vi "Locate SCM Breakdown.vi"(0 "Signals":waveform(dbl)[](array[waveform]), 7 "Offset (µs)":dbl format="%#_13g", 9 "Duration (µs)":dbl format="%#_13g", 11 "error in (no error)":errorcluster, 13 "Microphone Coordinates (cm, rad)":cluster{"r":dbl, "theta":dbl}[](array[cluster])) -> (4 "Coordinates (cm, rad, cm)":cluster{"r":sgl, "theta":sgl, "z":sgl}[](array[cluster]), 8 "Upstream/Downstream Delay (s)":dbl, 15 "error out":errorcluster)   [LabVIEW 2013]
uses:
  <vilib>/Analysis/2dsp.llb/1D Cross Correlation (DBL).vi
  <vilib>/Waveform/WDTOps.llb/WDT Get Waveform Subset DBL.vi
  <vilib>/Waveform/WDTOps.llb/WDT Index Channel DBL.vi
  <vilib>/Analysis/NI_AALPro.lvlib
  Breakdown Acoustics Controls/Breakdown Acoustics Controls.lvlib
panel:
  out "Sampling Rate":u16
  out "Array":i32[](array[numeric])
  out "Source Signals Correlation":dbl[](graph)
  out "Shifted Source Signals":dbl[][](graph)
  out "Downstream Signals":waveform(dbl)[](graph)
  out "Upstream Signals":waveform(dbl)[](graph)
  out "Duration (S)":dbl
  out "Offset (S)":dbl
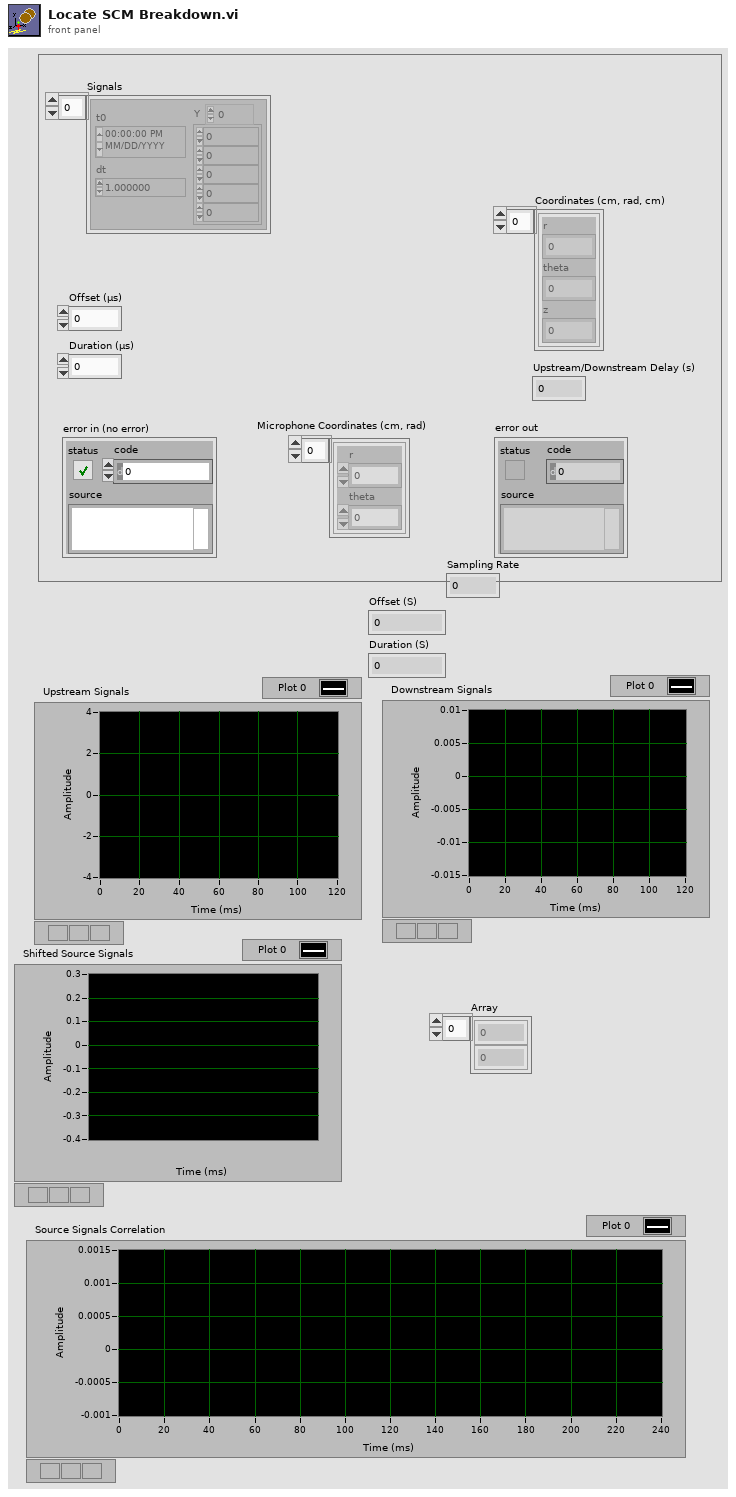
[diagram p1: front panel]
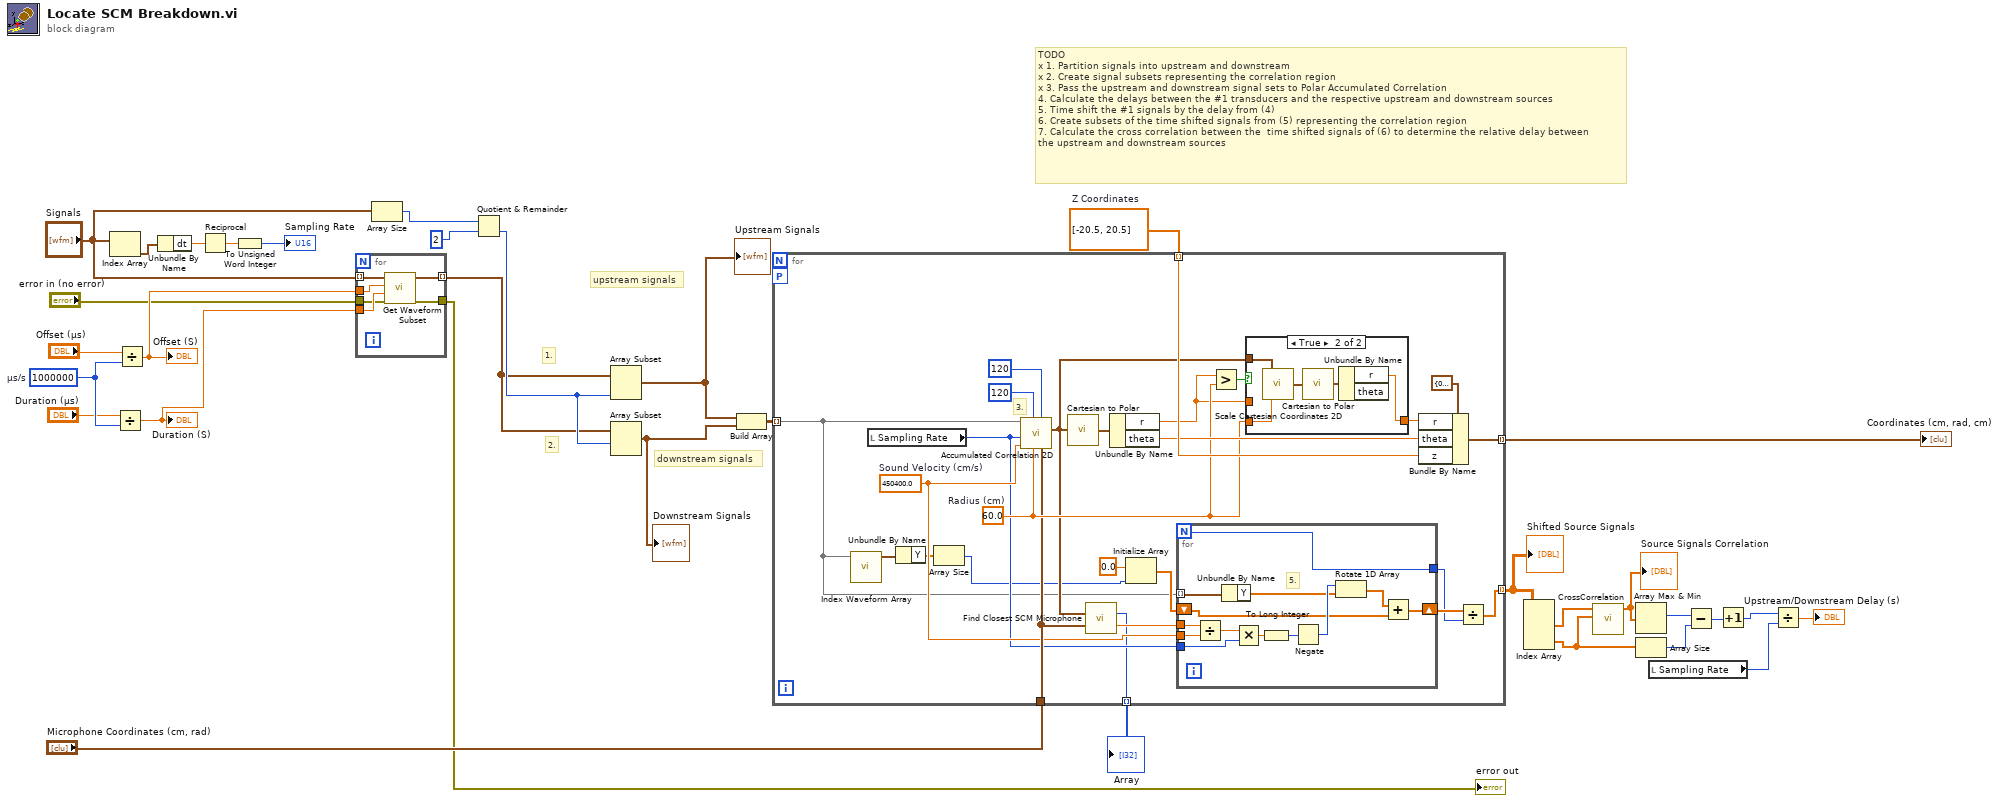
[diagram p0: block diagram]
diagram:
  w32 = dbl[] [-20.5, 20.5]  # Z Coordinates
  w7 = 1000000  # µs/s
  # "2."
  # "1."
  # "downstream signals"
  # "upstream signals"
  # "TODO\nx 1. Partition signals into upstream and downstream\nx 2. Create signal subsets representing the correlation region\nx 3. Pass the upstream and downstream signal sets to Polar Accumulated Correlation\n4. Calculate the delays between the #1 transducers and the respective upstream and downstream sources\n5. Time shift the #1 signals by the delay from (4)\n6. Create subsets of the time shifted signals from (5) representing the correlation region\n7. Calculate the cross correlation between the  time shifted signals of (6) to determine the relative delay between\nthe upstream and downstream sources"
  n1 = Index Array(array="Signals") -> (element=w9:waveform(dbl))  [unwired: 1 in]
  n2 = Divide(x="Duration (µs)", y=w7) -> (x/y=w13:dbl)
  "Duration (S)" <- w13
  n3 = Divide(x="Offset (µs)", y=w7) -> (x/y=w14:dbl)
  "Offset (S)" <- w14
  n4 = Unbundle By Name(w9) -> ("dt"=w8:dbl)
  n5 = Reciprocal(x=w8) -> (1/x=w2:dbl)
  n6 = To Unsigned Word Integer(number=w2) -> (unsigned 16bit integer=→"Sampling Rate":u16)
  n7 = for {
    tunnel: "Signals" -> [w39] mode=indexing
    tunnel: [w38] -> w15 mode=indexing
    tunnel: w14 -> [w37]
    tunnel: w13 -> [w36]
    tunnel: "error in (no error)" -> [w35]
    tunnel: [w34] -> w3
    n8 = call-poly <vilib>:"Get Waveform Subset.vi"("error in (no error)"=w35, "duration"=w36, "start samples/time"=w37, "waveform in"=w39) -> ("error out"=w34:errorcluster, "waveform out"=w38:waveform(dbl))  [unwired: 2 in, 2 out]
  }
  "error out" <- w3
  n9 = Array Size(array="Signals") -> (size(s)=w11:i32)
  n10 = Quotient & Remainder(x=w11, y=2) -> (floor(x/y)=w22:i32)  [unwired: 1 out]
  n11 = Array Subset(array=w15, length=w22) -> (w12:waveform(dbl)[])  [unwired: 1 in]
  "Upstream Signals" <- w12
  n12 = Array Subset(array=w15, index=w22) -> (w21:waveform(dbl)[])  [unwired: 1 in]
  "Downstream Signals" <- w21
  n13 = Build Array(w12, w21) -> (w33:waveform(dbl)[][])
  n14 = for {
    tunnel: w33 -> [w41] mode=indexing
    tunnel: "Microphone Coordinates (cm, rad)" -> [w53]
    tunnel: w32 -> [w63] mode=indexing
    tunnel: [w62] -> w25 mode=indexing
    tunnel: [w48] -> w18 mode=indexing
    workers-P: _ -> [_]
    tunnel: [w49] -> w16 mode=indexing
    w56 = 60.0  # Radius (cm)
    w51 = 450400.0  # Sound Velocity (cm/s)
    # "3."
    n15 = call-poly <vilib>:"Index Waveform Array.vi"("waveform array"=w41) -> ("waveform"=w43:waveform(dbl))  [unwired: 9 in, 1 out]
    n16 = local read "Sampling Rate"() -> (w50:u16)
    n17 = Unbundle By Name(w43) -> ("Y"=w42:dbl[])
    n18 = Array Size(array=w42) -> (size(s)=w40:i32)
    n19 = call "Accumulated Correlation 2D.vi"("Microphone Coordinates (cm, rad)"=w53, "Ny"=120 ("Ntheta"), "Radius (cm)"=w56, "Nx"=120 ("Nr"), "Sound Velocity (cm/s)"=w51, "Sampling Rate"=w50, "Waveforms"=w41) -> ("Source Coordinates (cm, cm)"=w54:cluster{"x":dbl, "y":dbl})  [unwired: 4 in]
    n20 = call "Cartesian to Polar.vi"("Cartesian\nCoordinates"=w54) -> ("Polar\nCoordinates"=w61:cluster{"r":dbl, "theta":dbl})  [unwired: 4 in]
    n21 = call "Find Closest SCM Microphone.vi"("Source Polar\nCoordinates"=w54, "Microphone Coordinates (cm, rad)"=w53) -> ("Closest Microphone Index"=w49:i32, "Closest Microphone Distance (cm)"=w52:dbl)  [unwired: 12 in]
    n22 = Unbundle By Name(w61) -> ("r"=w55:dbl, "theta"=w60:dbl)
    n23 = Initialize Array(0.0 ("element"), w40) -> (w44:dbl[])
    n24 = for {
      N -> [w69]
      tunnel: w52 -> [w78]
      tunnel: w51 -> [w77]
      tunnel: w50 -> [w75]
      tunnel: w41 -> [w67] mode=indexing
      shift-right: [w70] -> w47
      shift-left: w44 -> [w68]
      tunnel: [w69] -> w46
      # "5."
      n25 = Divide(x=w78, y=w77) -> (x/y=w76:dbl)
      n26 = Unbundle By Name(w67) -> ("Y"=w66:dbl[])
      n27 = Multiply(x=w76, y=w75) -> (x*y=w74:dbl)
      n28 = To Long Integer(number=w74) -> (32bit integer=w73:i32)
      n29 = Negate(x=w73) -> (-x=w72:i32)
      n30 = Rotate 1D Array(1:w66, 2:w72) -> (0:w71:dbl[])
      n31 = Add(x=w71, y=w68) -> (x+y=w70:dbl[])
    }
    n32 = Greater?(x=w55, y=w56) -> (0:w58:bool)
    n33 = case shown="True" w58 {
      tunnel: w56 -> [_ w83]
      tunnel: [w79 w80] -> w57
      tunnel: w54 -> [_ w84]
      tunnel: w55 -> [w79 _]
      frame False {
      }
      frame True {
        n34 = call "Scale Cartesian Coordinates 2D.vi"("Max Radius"=w83, "Source Coordinates (cm, cm)"=w84) -> ("output cluster"=w82:cluster{"x":dbl, "y":dbl})  [unwired: 3 in]
        n35 = call "Cartesian to Polar.vi"("Cartesian\nCoordinates"=w82) -> ("Polar\nCoordinates"=w81:cluster{"r":dbl, "theta":dbl})  [unwired: 4 in]
        n36 = Unbundle By Name(w81) -> ("r"=w80:dbl)  [unwired: 1 out]
      }
    }
    n37 = Bundle By Name(cluster=cluster{"r":sgl, "theta":sgl, "z":sgl} {"r"=0.0, "theta"=0.0, "z"=0.0} ("Coordinates (m)"), "r"=w57, "theta"=w60, "z"=w63) -> (w62:cluster{"r":sgl, "theta":sgl, "z":sgl})
    n38 = Divide(x=w47, y=w46) -> (x/y=w48:dbl[])
  }
  "Coordinates (cm, rad, cm)" <- w25
  "Shifted Source Signals" <- w18
  "Array" <- w16
  n39 = Index Array(array=w18) -> (element #1=w20:dbl[], element #2=w19:dbl[])  [unwired: 4 in]
  n40 = call-poly <vilib>:"CrossCorrelation.vi"("Y"=w19, "X"=w20) -> ("Rxy"=w17:dbl[])  [unwired: 8 in, 1 out]
  "Source Signals Correlation" <- w17
  n41 = Array Max & Min(array=w17) -> (max index (indices)=w31:i32)  [unwired: 3 out]
  n42 = Array Size ("Size(s)")(array=w19) -> (size(s)=w30:i32)
  n43 = local read "Sampling Rate"() -> (w27:u16)
  n44 = Subtract(x=w31, y=w30) -> (x-y=w29:i32)
  n45 = Increment(x=w29) -> (x+1=w28:i32)
  n46 = Divide(x=w28, y=w27) -> (x/y=→"Upstream/Downstream Delay (s)":dbl)
